vi "VectorNav Check.vi"() -> (0 "Vector Nav Check":bool)   [LabVIEW 2010]
uses:
  7.0-Global.vi
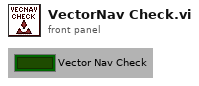
[diagram p1: front panel]
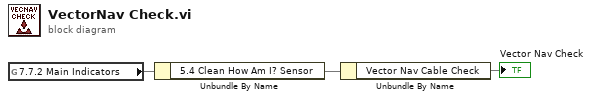
[diagram p0: block diagram]
diagram:
  n1 = global read "7.0-Global.vi" "7.7.2 Main Indicators"() -> (w3)
  n2 = Unbundle By Name(w3) -> ("5.4 Clean How Am I? Sensor"=w2)
  n3 = Unbundle By Name(w2) -> ("Vector Nav Cable Check"=→"Vector Nav Check")
